vi "Create 4 In 4 Out Channel Resources.vi"(0 "common resources":T1={"sync pulse resources"={"sync pulse destination terminal"="", "sync100"="", "sync pulse source terminal"="", "imported sync pulse register"="", "generate sync pulse handshake"="", "enable sync pulse register"="", "sync pulse clock"=""}, "serial channel resources"={"sc 0"={"completed frames register"=""}, "sc 1"={"completed frames register"=""}, "sc 2"={"completed frames register"=""}, "sc 3"={"completed frames register"=""}, "sc 4"={"completed frames register"=""}, "sc 5"={"completed frames register"=""}, "sc 6"={"completed frames register"=""}, "sc 7"={"completed frames register"=""}}, "dram manager 0"={"DRAM class"=refnum, "process clock"="", "registers"={"configuration"={"write time slice"="", "request time slice"="", "DRAM arbiter config"="", "partition config"=""}, "reset"={"handshake"={"start.go"="", "start.go rcvd"="", "done.go"="", "done.go rcvd"=""}, "process"={"in"="", "out"=""}, "write"={"in"="", "out 0"="", "out 1"="", "out 2"="", "out 3"=""}, "read"={"in"="", "out 0"="", "out 1"="", "out 2"="", "out 3"=""}}, "status"={"partition full"=""}}, "FIFOs"={"write data"={"FIFO 0"="", "FIFO 1"="", "FIFO 2"="", "FIFO 3"=""}, "request metadata"={"FIFO"=""}, "read data VOQ"={"FIFO 0"="", "FIFO 1"="", "FIFO 2"="", "FIFO 3"=""}, "read data"={"FIFO 0"="", "FIFO 1"="", "FIFO 2"="", "FIFO 3"=""}}, "num active streams"=0.0, "max open read requests"=256}, "dram manager 1"={"DRAM class"=refnum, "process clock"="", "registers"={"configuration"={"write time slice"="", "request time slice"="", "DRAM arbiter config"="", "partition config"=""}, "reset"={"handshake"={"start.go"="", "start.go rcvd"="", "done.go"="", "done.go rcvd"=""}, "process"={"in"="", "out"=""}, "write"={"in"="", "out 0"="", "out 1"="", "out 2"="", "out 3"=""}, "read"={"in"="", "out 0"="", "out 1"="", "out 2"="", "out 3"=""}}, "status"={"partition full"=""}}, "FIFOs"={"write data"={"FIFO 0"="", "FIFO 1"="", "FIFO 2"="", "FIFO 3"=""}, "request metadata"={"FIFO"=""}, "read data VOQ"={"FIFO 0"="", "FIFO 1"="", "FIFO 2"="", "FIFO 3"=""}, "read data"={"FIFO 0"="", "FIFO 1"="", "FIFO 2"="", "FIFO 3"=""}}, "num active streams"=0.0, "max open read requests"=256}}, 5 "dram partition configs":T12[](array[typedef])=[{"first address"=0, "last address"=0}, {"first address"=0, "last address"=0}, {"first address"=0, "last address"=0}, {"first address"=0, "last address"=0}, {"first address"=0, "last address"=0}, {"first address"=0, "last address"=0}, {"first address"=0, "last address"=0}, {"first address"=0, "last address"=0}]) -> (4 "channel resources":T13)   [LabVIEW 2020, in "GettingStarted_Acq_Tap_148X_FPGA.lvlib"]
uses:
  GettingStarted_Acq_Tap_148X_FPGA.lvlib
  Types/4 In 4 Out Channel Resources.ctl
  <instrlib>/_niInstr/Memory/v1/FPGA/DRAM/niInstr Memory DRAM v1 FPGA.lvclass
  Types/Serial Input Channel Resources.ctl
  <instrlib>/FlexRIO/CSI-2/v2/FPGA/DRAM Manager/Private/DRAM Manager.ctl
  <instrlib>/FlexRIO/CSI-2/v2/FPGA/DRAM Manager/Private/Common/DRAM Manager Registers.ctl
  <instrlib>/FlexRIO/CSI-2/v2/FPGA/DRAM Manager/Private/Common/Handshake Registers.ctl
  <instrlib>/FlexRIO/CSI-2/v2/FPGA/DRAM Manager/Private/Common/DRAM Manager FIFOs.ctl
  <instrlib>/FlexRIO/CSI-2/v2/FPGA/DRAM Manager/Private/Common/Write Data FIFO Ref.ctl
  <instrlib>/FlexRIO/CSI-2/v2/FPGA/DRAM Manager/Private/Common/Read Request Metadata FIFO Ref.ctl
  <instrlib>/FlexRIO/CSI-2/v2/FPGA/DRAM Manager/Private/Common/Read Data FIFO Ref.ctl
  Types/Serial Input Channel IO.ctl
  Types/Serial Input Channel IO 32b.ctl
  Types/Serial Input Channel IO 64b.ctl
  Common/Types/I2C IO.ctl
  Types/Serial Ouput Channel Resources.ctl
  Common/Types/Serial Output Channel IO.ctl
  Common/Types/Serial Output Channel IO 32b.ctl
  Common/Types/Serial Output Channel IO 64b.ctl
  <instrlib>/FlexRIO/CSI-2/v2/FPGA/DRAM Manager/Public/Partition Range.ctl
  Common/Types/Common Resources.ctl
  <instrlib>/FlexRIO/CSI-2/v2/FPGA/Types/Sync Pulse Resources.ctl
  Common/Types/Serial Channel Resources.ctl
  Common/Types/Single Serial Channel Resources.ctl
  <instrlib>/FlexRIO/CSI-2/v2/FPGA/DRAM Manager/DRAM Manager v2.lvlib
  Common/GettingStarted_Common_148X_FPGA.lvlib
  <instrlib>/FlexRIO/CSI-2/v2/FPGA/NI CSI-2 API FPGA v2.lvlib
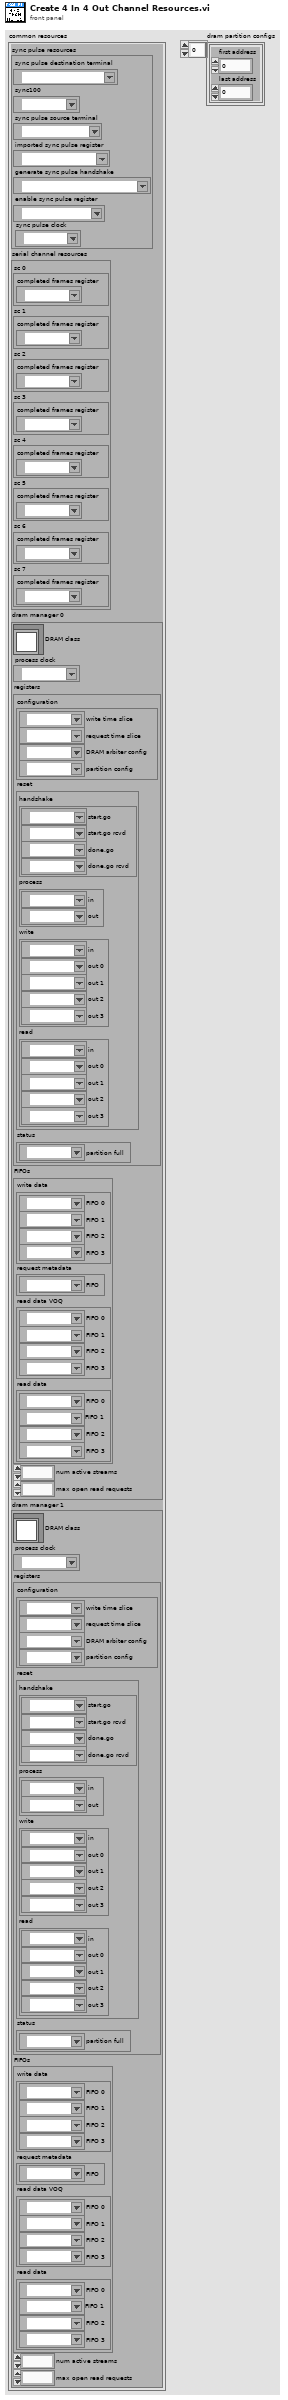
[diagram p1: front panel]
types:
  T1 = typedef "GettingStarted_Common_148X_FPGA.lvlib/Common Resources.ctl" = cluster{"sync pulse resources":T2, "serial channel resources":T3, "dram manager 0":T5, "dram manager 1":T5}
  T2 = typedef "NI CSI-2 API FPGA v2.lvlib/Sync Pulse Resources.ctl" = cluster{"sync pulse destination terminal":refnum<k21>, "sync100":refnum<k21>, "sync pulse source terminal":refnum<k21>, "imported sync pulse register":refnum<k21>, "generate sync pulse handshake":refnum<k21>, "enable sync pulse register":refnum<k21>, "sync pulse clock":refnum<k21>}
  T3 = typedef "GettingStarted_Common_148X_FPGA.lvlib/Serial Channel Resources.ctl" = cluster{"sc 0":T4, "sc 1":T4, "sc 2":T4, "sc 3":T4, "sc 4":T4, "sc 5":T4, "sc 6":T4, "sc 7":T4}
  T4 = typedef "GettingStarted_Common_148X_FPGA.lvlib/Single Serial Channel Resources.ctl" = cluster{"completed frames register":refnum<k21>}
  T5 = typedef "DRAM Manager v2.lvlib/DRAM Manager.ctl" = cluster{"DRAM class":refnum<class "niInstr Memory DRAM v1 FPGA.lvclass">, "process clock":refnum<k21>, "registers":T6, "FIFOs":T8, "num active streams":fxp<+,3,3>, "max open read requests":u16}
  T6 = typedef "DRAM Manager v2.lvlib/DRAM Manager Registers.ctl" = cluster{"configuration":cluster{"write time slice":refnum<k21>, "request time slice":refnum<k21>, "DRAM arbiter config":refnum<k21>, "partition config":refnum<k21>}, "reset":cluster{"handshake":T7, "process":cluster{"in":refnum<k21>, "out":refnum<k21>}, "write":cluster{"in":refnum<k21>, "out 0":refnum<k21>, "out 1":refnum<k21>, "out 2":refnum<k21>, "out 3":refnum<k21>}, "read":cluster{"in":refnum<k21>, "out 0":refnum<k21>, "out 1":refnum<k21>, "out 2":refnum<k21>, "out 3":refnum<k21>}}, "status":cluster{"partition full":refnum<k21>}}
  T7 = typedef "DRAM Manager v2.lvlib/Handshake Registers.ctl" = cluster{"start.go":refnum<k21>, "start.go rcvd":refnum<k21>, "done.go":refnum<k21>, "done.go rcvd":refnum<k21>}
  T8 = typedef "DRAM Manager v2.lvlib/DRAM Manager FIFOs.ctl" = cluster{"write data":cluster{"FIFO 0":T9, "FIFO 1":T9, "FIFO 2":T9, "FIFO 3":T9}, "request metadata":cluster{"FIFO":T10}, "read data VOQ":cluster{"FIFO 0":T11, "FIFO 1":T11, "FIFO 2":T11, "FIFO 3":T11}, "read data":cluster{"FIFO 0":T11, "FIFO 1":T11, "FIFO 2":T11, "FIFO 3":T11}}
  T9 = typedef "DRAM Manager v2.lvlib/Write Data FIFO Ref.ctl" = refnum<k21>
  T10 = typedef "DRAM Manager v2.lvlib/Read Request Metadata FIFO Ref.ctl" = refnum<k21>
  T11 = typedef "DRAM Manager v2.lvlib/Read Data FIFO Ref.ctl" = refnum<k21>
  T12 = typedef "DRAM Manager v2.lvlib/Partition Range.ctl" = cluster{"first address":u32, "last address":u32}
  T13 = typedef "GettingStarted_Acq_Tap_148X_FPGA.lvlib/4 In 4 Out Channel Resources.ctl" = cluster{"si 0 resources":T14, "si 1 resources":T14, "si 2 resources":T14, "si 3 resources":T14, "so 0 resources":T19, "so 1 resources":T19, "so 2 resources":T19, "so 3 resources":T19}
  T14 = typedef "GettingStarted_Acq_Tap_148X_FPGA.lvlib/Serial Input Channel Resources.ctl" = cluster{"dram manager":T5, "csi-2 input io":T15, "serial input channel instance":u8, "dram stream id":fxp<+,2,2>, "i2c io":T18}
  T15 = typedef "GettingStarted_Acq_Tap_148X_FPGA.lvlib/Serial Input Channel IO.ctl" = cluster{"32b":T16, "64b":T17, "csi-2 axi stream tlast":refnum<k21>, "csi-2 axi stream tvalid":refnum<k21>}
  T16 = typedef "GettingStarted_Acq_Tap_148X_FPGA.lvlib/Serial Input Channel IO 32b.ctl" = cluster{"csi-2 axi stream tdata":refnum<k21>, "csi-2 axi stream raw tdata":refnum<k21>, "csi-2 axi stream tuser":refnum<k21>}
  T17 = typedef "GettingStarted_Acq_Tap_148X_FPGA.lvlib/Serial Input Channel IO 64b.ctl" = cluster{"csi-2 axi stream tdata":refnum<k21>, "csi-2 axi stream raw tdata":refnum<k21>, "csi-2 axi stream tuser":refnum<k21>}
  T18 = typedef "GettingStarted_Common_148X_FPGA.lvlib/I2C IO.ctl" = cluster{"sda input":refnum<k21>, "sda output enable":refnum<k21>, "scl input":refnum<k21>, "scl output enable":refnum<k21>}
  T19 = typedef "GettingStarted_Acq_Tap_148X_FPGA.lvlib/Serial Ouput Channel Resources.ctl" = cluster{"csi-2 output io":T20, "i2c io":T18}
  T20 = typedef "GettingStarted_Common_148X_FPGA.lvlib/Serial Output Channel IO.ctl" = cluster{"32b":T21, "64b":T22, "csi-2 axi stream tready":refnum<k21>, "csi-2 axi stream tvalid":refnum<k21>, "csi-2 axi stream tlast":refnum<k21>, "num packets in tx fifo":refnum<k21>, "ready to transmit packet":refnum<k21>, "transmit packet done":refnum<k21>, "transmit packet":refnum<k21>}
  T21 = typedef "GettingStarted_Common_148X_FPGA.lvlib/Serial Output Channel IO 32b.ctl" = cluster{"csi-2 axi stream tdata":refnum<k21>, "csi-2 axi stream tuser":refnum<k21>}
  T22 = typedef "GettingStarted_Common_148X_FPGA.lvlib/Serial Output Channel IO 64b.ctl" = cluster{"csi-2 axi stream tdata":refnum<k21>, "csi-2 axi stream tuser":refnum<k21>}
  T23 = cluster{"serial input 0 csi-2 io":T15, "serial input 1 csi-2 io":T15, "serial input 2 csi-2 io":T15, "serial input 3 csi-2 io":T15}
  T24 = cluster{"serial input 0 i2c io":T18, "serial input 1 i2c io":T18, "serial input 2 i2c io":T18, "serial input 3 i2c io":T18}
  T25 = cluster{"serial output 0 io":T20, "serial output 1 io":T20, "serial output 2 io":T20, "serial output 3 io":T20}
  T26 = cluster{"serial output 2 i2c io":T18, "serial output 1 i2c io":T18, "serial output 0 i2c io":T18, "serial output 3 i2c io":T18}
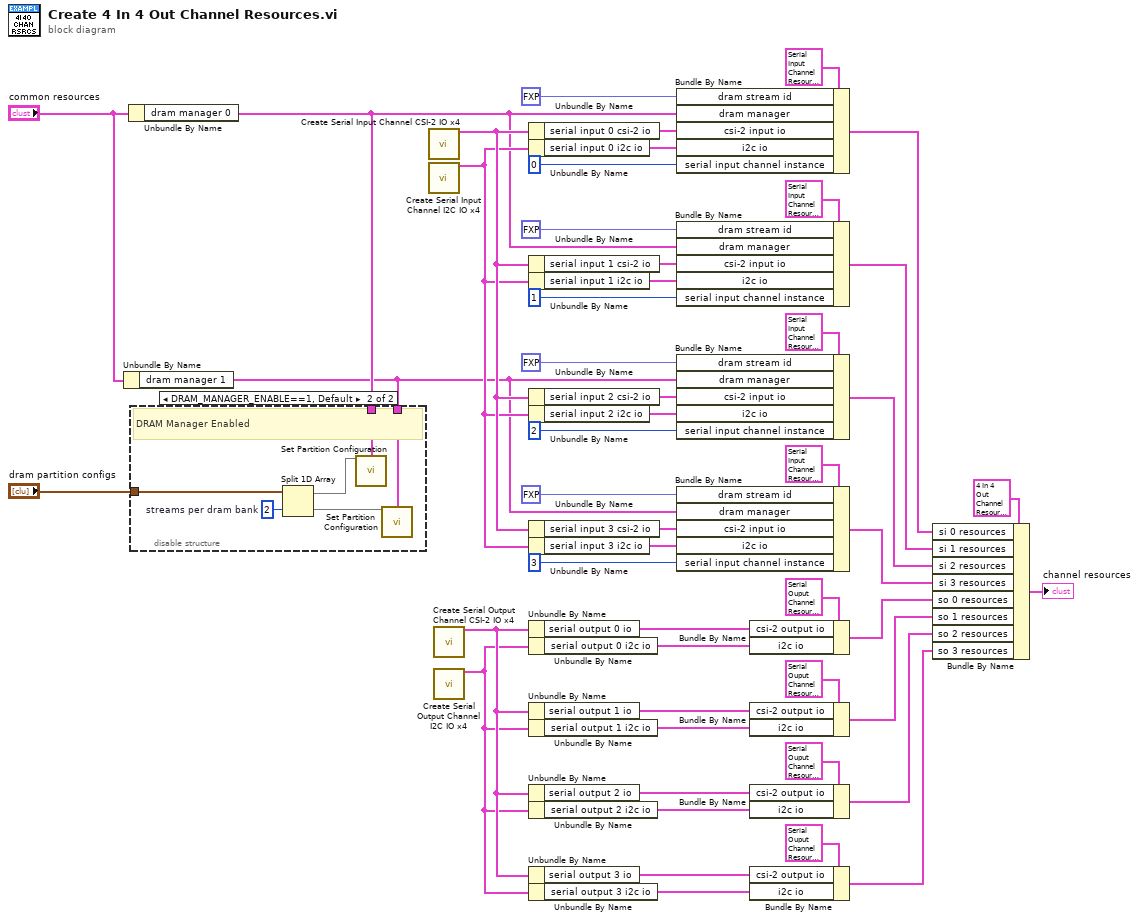
[diagram p0: block diagram]
diagram:
  n1 = Unbundle By Name("common resources") -> ("dram manager 1"=w3:T5)
  n2 = Unbundle By Name("common resources") -> ("dram manager 0"=w4:T5)
  n3 = disable-structure shown="DRAM_MANAGER_ENABLE==1, Default" {
    disable-tunnel: w4 -> [_ w53]
    disable-tunnel: w3 -> [_ w52]
    disable-tunnel: "dram partition configs" -> [_ w51]
    frame condition #0 {
      # "DRAM Manager Disabled"
    }
    frame condition #1 (active) {
      w56 = 2  # streams per dram bank
      # "DRAM Manager Enabled"
      n4 = Split 1D Array(array=w51, index=w56) -> (first subarray=w55:T12[], second subarray=w54:T12[])
      n5 = call <instrlib>:"Set Partition Configuration.vi"("partition config"=w55, "DRAM manager"=w53) -> ()  [unwired: 14 in]
      n6 = call <instrlib>:"Set Partition Configuration.vi"("partition config"=w54, "DRAM manager"=w52) -> ()  [unwired: 14 in]
    }
  }
  n7 = call "Create Serial Input Channel CSI-2 IO x4.vi"() -> ("serial input csi-2 io x4"=w20:T23)  [unwired: 15 in]
  n8 = call "Create Serial Input Channel I2C IO x4.vi"() -> ("serial input channel i2c io x4"=w5:T24)  [unwired: 15 in]
  n9 = call "Create Serial Output Channel CSI-2 IO x4.vi"() -> ("serial output channel csi-2 io x4 2"=w15:T25)  [unwired: 15 in]
  n10 = call "Create Serial Output Channel I2C IO x4.vi"() -> ("serial output channel i2c io x4"=w10:T26)  [unwired: 15 in]
  n11 = Unbundle By Name(w20) -> ("serial input 0 csi-2 io"=w24:T15)
  n12 = Unbundle By Name(w5) -> ("serial input 0 i2c io"=w6:T18)
  n13 = Unbundle By Name(w20) -> ("serial input 1 csi-2 io"=w23:T15)
  n14 = Unbundle By Name(w5) -> ("serial input 1 i2c io"=w7:T18)
  n15 = Unbundle By Name(w20) -> ("serial input 2 csi-2 io"=w22:T15)
  n16 = Unbundle By Name(w5) -> ("serial input 2 i2c io"=w8:T18)
  n17 = Unbundle By Name(w20) -> ("serial input 3 csi-2 io"=w21:T15)
  n18 = Unbundle By Name(w5) -> ("serial input 3 i2c io"=w9:T18)
  n19 = Unbundle By Name(w15) -> ("serial output 0 io"=w19:T20)
  n20 = Unbundle By Name(w10) -> ("serial output 0 i2c io"=w14:T18)
  n21 = Unbundle By Name(w15) -> ("serial output 1 io"=w18:T20)
  n22 = Unbundle By Name(w10) -> ("serial output 1 i2c io"=w13:T18)
  n23 = Unbundle By Name(w15) -> ("serial output 2 io"=w17:T20)
  n24 = Unbundle By Name(w10) -> ("serial output 2 i2c io"=w12:T18)
  n25 = Unbundle By Name(w15) -> ("serial output 3 io"=w16:T20)
  n26 = Unbundle By Name(w10) -> ("serial output 3 i2c io"=w11:T18)
  n27 = Bundle By Name(cluster=T14 {"dram manager"={"DRAM class"=refnum, "process clock"="", "registers"={"configuration"={"write time slice"="", "request time slice"="", "DRAM arbiter config"="", "partition config"=""}, "reset"={"handshake"={"start.go"="", "start.go rcvd"="", "done.go"="", "done.go rcvd"=""}, "process"={"in"="", "out"=""}, "write"={"in"="", "out 0"="", "out 1"="", "out 2"="", "out 3"=""}, "read"={"in"="", "out 0"="", "out 1"="", "out 2"="", "out 3"=""}}, "status"={"partition full"=""}}, "FIFOs"={"write data"={"FIFO 0"="", "FIFO 1"="", "FIFO 2"="", "FIFO 3"=""}, "request metadata"={"FIFO"=""}, "read data VOQ"={"FIFO 0"="", "FIFO 1"="", "FIFO 2"="", "FIFO 3"=""}, "read data"={"FIFO 0"="", "FIFO 1"="", "FIFO 2"="", "FIFO 3"=""}}, "num active streams"=0.0, "max open read requests"=0}, "csi-2 input io"={"32b"={"csi-2 axi stream tdata"="", "csi-2 axi stream raw tdata"="", "csi-2 axi stream tuser"=""}, "64b"={"csi-2 axi stream tdata"="", "csi-2 axi stream raw tdata"="", "csi-2 axi stream tuser"=""}, "csi-2 axi stream tlast"="", "csi-2 axi stream tvalid"=""}, "serial input channel instance"=0, "dram stream id"=0.0, "i2c io"={"sda input"="", "sda output enable"="", "scl input"="", "scl output enable"=""}} ("si 0 resources"), "dram stream id"=fxp<+,2,2> 0.0, "dram manager"=w4, "csi-2 input io"=w24, "i2c io"=w6, "serial input channel instance"=u8 0) -> (w50:T14)
  n28 = Bundle By Name(cluster=T14 {"dram manager"={"DRAM class"=refnum, "process clock"="", "registers"={"configuration"={"write time slice"="", "request time slice"="", "DRAM arbiter config"="", "partition config"=""}, "reset"={"handshake"={"start.go"="", "start.go rcvd"="", "done.go"="", "done.go rcvd"=""}, "process"={"in"="", "out"=""}, "write"={"in"="", "out 0"="", "out 1"="", "out 2"="", "out 3"=""}, "read"={"in"="", "out 0"="", "out 1"="", "out 2"="", "out 3"=""}}, "status"={"partition full"=""}}, "FIFOs"={"write data"={"FIFO 0"="", "FIFO 1"="", "FIFO 2"="", "FIFO 3"=""}, "request metadata"={"FIFO"=""}, "read data VOQ"={"FIFO 0"="", "FIFO 1"="", "FIFO 2"="", "FIFO 3"=""}, "read data"={"FIFO 0"="", "FIFO 1"="", "FIFO 2"="", "FIFO 3"=""}}, "num active streams"=0.0, "max open read requests"=0}, "csi-2 input io"={"32b"={"csi-2 axi stream tdata"="", "csi-2 axi stream raw tdata"="", "csi-2 axi stream tuser"=""}, "64b"={"csi-2 axi stream tdata"="", "csi-2 axi stream raw tdata"="", "csi-2 axi stream tuser"=""}, "csi-2 axi stream tlast"="", "csi-2 axi stream tvalid"=""}, "serial input channel instance"=0, "dram stream id"=0.0, "i2c io"={"sda input"="", "sda output enable"="", "scl input"="", "scl output enable"=""}} ("si 0 resources"), "dram stream id"=fxp<+,2,2> 1.0, "dram manager"=w4, "csi-2 input io"=w23, "i2c io"=w7, "serial input channel instance"=u8 1) -> (w49:T14)
  n29 = Bundle By Name(cluster=T14 {"dram manager"={"DRAM class"=refnum, "process clock"="", "registers"={"configuration"={"write time slice"="", "request time slice"="", "DRAM arbiter config"="", "partition config"=""}, "reset"={"handshake"={"start.go"="", "start.go rcvd"="", "done.go"="", "done.go rcvd"=""}, "process"={"in"="", "out"=""}, "write"={"in"="", "out 0"="", "out 1"="", "out 2"="", "out 3"=""}, "read"={"in"="", "out 0"="", "out 1"="", "out 2"="", "out 3"=""}}, "status"={"partition full"=""}}, "FIFOs"={"write data"={"FIFO 0"="", "FIFO 1"="", "FIFO 2"="", "FIFO 3"=""}, "request metadata"={"FIFO"=""}, "read data VOQ"={"FIFO 0"="", "FIFO 1"="", "FIFO 2"="", "FIFO 3"=""}, "read data"={"FIFO 0"="", "FIFO 1"="", "FIFO 2"="", "FIFO 3"=""}}, "num active streams"=0.0, "max open read requests"=0}, "csi-2 input io"={"32b"={"csi-2 axi stream tdata"="", "csi-2 axi stream raw tdata"="", "csi-2 axi stream tuser"=""}, "64b"={"csi-2 axi stream tdata"="", "csi-2 axi stream raw tdata"="", "csi-2 axi stream tuser"=""}, "csi-2 axi stream tlast"="", "csi-2 axi stream tvalid"=""}, "serial input channel instance"=0, "dram stream id"=0.0, "i2c io"={"sda input"="", "sda output enable"="", "scl input"="", "scl output enable"=""}} ("si 0 resources"), "dram stream id"=fxp<+,2,2> 0.0, "dram manager"=w3, "csi-2 input io"=w22, "i2c io"=w8, "serial input channel instance"=u8 2) -> (w48:T14)
  n30 = Bundle By Name(cluster=T14 {"dram manager"={"DRAM class"=refnum, "process clock"="", "registers"={"configuration"={"write time slice"="", "request time slice"="", "DRAM arbiter config"="", "partition config"=""}, "reset"={"handshake"={"start.go"="", "start.go rcvd"="", "done.go"="", "done.go rcvd"=""}, "process"={"in"="", "out"=""}, "write"={"in"="", "out 0"="", "out 1"="", "out 2"="", "out 3"=""}, "read"={"in"="", "out 0"="", "out 1"="", "out 2"="", "out 3"=""}}, "status"={"partition full"=""}}, "FIFOs"={"write data"={"FIFO 0"="", "FIFO 1"="", "FIFO 2"="", "FIFO 3"=""}, "request metadata"={"FIFO"=""}, "read data VOQ"={"FIFO 0"="", "FIFO 1"="", "FIFO 2"="", "FIFO 3"=""}, "read data"={"FIFO 0"="", "FIFO 1"="", "FIFO 2"="", "FIFO 3"=""}}, "num active streams"=0.0, "max open read requests"=0}, "csi-2 input io"={"32b"={"csi-2 axi stream tdata"="", "csi-2 axi stream raw tdata"="", "csi-2 axi stream tuser"=""}, "64b"={"csi-2 axi stream tdata"="", "csi-2 axi stream raw tdata"="", "csi-2 axi stream tuser"=""}, "csi-2 axi stream tlast"="", "csi-2 axi stream tvalid"=""}, "serial input channel instance"=0, "dram stream id"=0.0, "i2c io"={"sda input"="", "sda output enable"="", "scl input"="", "scl output enable"=""}} ("si 0 resources"), "dram stream id"=fxp<+,2,2> 1.0, "dram manager"=w3, "csi-2 input io"=w21, "i2c io"=w9, "serial input channel instance"=u8 3) -> (w47:T14)
  n31 = Bundle By Name(cluster=T19 {"csi-2 output io"={"32b"={"csi-2 axi stream tdata"="", "csi-2 axi stream tuser"=""}, "64b"={"csi-2 axi stream tdata"="", "csi-2 axi stream tuser"=""}, "csi-2 axi stream tready"="", "csi-2 axi stream tvalid"="", "csi-2 axi stream tlast"="", "num packets in tx fifo"="", "ready to transmit packet"="", "transmit packet done"="", "transmit packet"=""}, "i2c io"={"sda input"="", "sda output enable"="", "scl input"="", "scl output enable"=""}} ("so 0 resources"), "csi-2 output io"=w19, "i2c io"=w14) -> (w46:T19)
  n32 = Bundle By Name(cluster=T19 {"csi-2 output io"={"32b"={"csi-2 axi stream tdata"="", "csi-2 axi stream tuser"=""}, "64b"={"csi-2 axi stream tdata"="", "csi-2 axi stream tuser"=""}, "csi-2 axi stream tready"="", "csi-2 axi stream tvalid"="", "csi-2 axi stream tlast"="", "num packets in tx fifo"="", "ready to transmit packet"="", "transmit packet done"="", "transmit packet"=""}, "i2c io"={"sda input"="", "sda output enable"="", "scl input"="", "scl output enable"=""}} ("so 0 resources"), "csi-2 output io"=w18, "i2c io"=w13) -> (w45:T19)
  n33 = Bundle By Name(cluster=T19 {"csi-2 output io"={"32b"={"csi-2 axi stream tdata"="", "csi-2 axi stream tuser"=""}, "64b"={"csi-2 axi stream tdata"="", "csi-2 axi stream tuser"=""}, "csi-2 axi stream tready"="", "csi-2 axi stream tvalid"="", "csi-2 axi stream tlast"="", "num packets in tx fifo"="", "ready to transmit packet"="", "transmit packet done"="", "transmit packet"=""}, "i2c io"={"sda input"="", "sda output enable"="", "scl input"="", "scl output enable"=""}} ("so 0 resources"), "csi-2 output io"=w17, "i2c io"=w12) -> (w44:T19)
  n34 = Bundle By Name(cluster=T19 {"csi-2 output io"={"32b"={"csi-2 axi stream tdata"="", "csi-2 axi stream tuser"=""}, "64b"={"csi-2 axi stream tdata"="", "csi-2 axi stream tuser"=""}, "csi-2 axi stream tready"="", "csi-2 axi stream tvalid"="", "csi-2 axi stream tlast"="", "num packets in tx fifo"="", "ready to transmit packet"="", "transmit packet done"="", "transmit packet"=""}, "i2c io"={"sda input"="", "sda output enable"="", "scl input"="", "scl output enable"=""}} ("so 0 resources"), "csi-2 output io"=w16, "i2c io"=w11) -> (w43:T19)
  n35 = Bundle By Name(cluster=T13 {"si 0 resources"={"dram manager"={"DRAM class"=refnum, "process clock"="", "registers"={"configuration"={"write time slice"="", "request time slice"="", "DRAM arbiter config"="", "partition config"=""}, "reset"={"handshake"={"start.go"="", "start.go rcvd"="", "done.go"="", "done.go rcvd"=""}, "process"={"in"="", "out"=""}, "write"={"in"="", "out 0"="", "out 1"="", "out 2"="", "out 3"=""}, "read"={"in"="", "out 0"="", "out 1"="", "out 2"="", "out 3"=""}}, "status"={"partition full"=""}}, "FIFOs"={"write data"={"FIFO 0"="", "FIFO 1"="", "FIFO 2"="", "FIFO 3"=""}, "request metadata"={"FIFO"=""}, "read data VOQ"={"FIFO 0"="", "FIFO 1"="", "FIFO 2"="", "FIFO 3"=""}, "read data"={"FIFO 0"="", "FIFO 1"="", "FIFO 2"="", "FIFO 3"=""}}, "num active streams"=0.0, "max open read requests"=0}, "csi-2 input io"={"32b"={"csi-2 axi stream tdata"="", "csi-2 axi stream raw tdata"="", "csi-2 axi stream tuser"=""}, "64b"={"csi-2 axi stream tdata"="", "csi-2 axi stream raw tdata"="", "csi-2 axi stream tuser"=""}, "csi-2 axi stream tlast"="", "csi-2 axi stream tvalid"=""}, "serial input channel instance"=0, "dram stream id"=0.0, "i2c io"={"sda input"="", "sda output enable"="", "scl input"="", "scl output enable"=""}}, "si 1 resources"={"dram manager"={"DRAM class"=refnum, "process clock"="", "registers"={"configuration"={"write time slice"="", "request time slice"="", "DRAM arbiter config"="", "partition config"=""}, "reset"={"handshake"={"start.go"="", "start.go rcvd"="", "done.go"="", "done.go rcvd"=""}, "process"={"in"="", "out"=""}, "write"={"in"="", "out 0"="", "out 1"="", "out 2"="", "out 3"=""}, "read"={"in"="", "out 0"="", "out 1"="", "out 2"="", "out 3"=""}}, "status"={"partition full"=""}}, "FIFOs"={"write data"={"FIFO 0"="", "FIFO 1"="", "FIFO 2"="", "FIFO 3"=""}, "request metadata"={"FIFO"=""}, "read data VOQ"={"FIFO 0"="", "FIFO 1"="", "FIFO 2"="", "FIFO 3"=""}, "read data"={"FIFO 0"="", "FIFO 1"="", "FIFO 2"="", "FIFO 3"=""}}, "num active streams"=0.0, "max open read requests"=0}, "csi-2 input io"={"32b"={"csi-2 axi stream tdata"="", "csi-2 axi stream raw tdata"="", "csi-2 axi stream tuser"=""}, "64b"={"csi-2 axi stream tdata"="", "csi-2 axi stream raw tdata"="", "csi-2 axi stream tuser"=""}, "csi-2 axi stream tlast"="", "csi-2 axi stream tvalid"=""}, "serial input channel instance"=0, "dram stream id"=0.0, "i2c io"={"sda input"="", "sda output enable"="", "scl input"="", "scl output enable"=""}}, "si 2 resources"={"dram manager"={"DRAM class"=refnum, "process clock"="", "registers"={"configuration"={"write time slice"="", "request time slice"="", "DRAM arbiter config"="", "partition config"=""}, "reset"={"handshake"={"start.go"="", "start.go rcvd"="", "done.go"="", "done.go rcvd"=""}, "process"={"in"="", "out"=""}, "write"={"in"="", "out 0"="", "out 1"="", "out 2"="", "out 3"=""}, "read"={"in"="", "out 0"="", "out 1"="", "out 2"="", "out 3"=""}}, "status"={"partition full"=""}}, "FIFOs"={"write data"={"FIFO 0"="", "FIFO 1"="", "FIFO 2"="", "FIFO 3"=""}, "request metadata"={"FIFO"=""}, "read data VOQ"={"FIFO 0"="", "FIFO 1"="", "FIFO 2"="", "FIFO 3"=""}, "read data"={"FIFO 0"="", "FIFO 1"="", "FIFO 2"="", "FIFO 3"=""}}, "num active streams"=0.0, "max open read requests"=0}, "csi-2 input io"={"32b"={"csi-2 axi stream tdata"="", "csi-2 axi stream raw tdata"="", "csi-2 axi stream tuser"=""}, "64b"={"csi-2 axi stream tdata"="", "csi-2 axi stream raw tdata"="", "csi-2 axi stream tuser"=""}, "csi-2 axi stream tlast"="", "csi-2 axi stream tvalid"=""}, "serial input channel instance"=0, "dram stream id"=0.0, "i2c io"={"sda input"="", "sda output enable"="", "scl input"="", "scl output enable"=""}}, "si 3 resources"={"dram manager"={"DRAM class"=refnum, "process clock"="", "registers"={"configuration"={"write time slice"="", "request time slice"="", "DRAM arbiter config"="", "partition config"=""}, "reset"={"handshake"={"start.go"="", "start.go rcvd"="", "done.go"="", "done.go rcvd"=""}, "process"={"in"="", "out"=""}, "write"={"in"="", "out 0"="", "out 1"="", "out 2"="", "out 3"=""}, "read"={"in"="", "out 0"="", "out 1"="", "out 2"="", "out 3"=""}}, "status"={"partition full"=""}}, "FIFOs"={"write data"={"FIFO 0"="", "FIFO 1"="", "FIFO 2"="", "FIFO 3"=""}, "request metadata"={"FIFO"=""}, "read data VOQ"={"FIFO 0"="", "FIFO 1"="", "FIFO 2"="", "FIFO 3"=""}, "read data"={"FIFO 0"="", "FIFO 1"="", "FIFO 2"="", "FIFO 3"=""}}, "num active streams"=0.0, "max open read requests"=0}, "csi-2 input io"={"32b"={"csi-2 axi stream tdata"="", "csi-2 axi stream raw tdata"="", "csi-2 axi stream tuser"=""}, "64b"={"csi-2 axi stream tdata"="", "csi-2 axi stream raw tdata"="", "csi-2 axi stream tuser"=""}, "csi-2 axi stream tlast"="", "csi-2 axi stream tvalid"=""}, "serial input channel instance"=0, "dram stream id"=0.0, "i2c io"={"sda input"="", "sda output enable"="", "scl input"="", "scl output enable"=""}}, "so 0 resources"={"csi-2 output io"={"32b"={"csi-2 axi stream tdata"="", "csi-2 axi stream tuser"=""}, "64b"={"csi-2 axi stream tdata"="", "csi-2 axi stream tuser"=""}, "csi-2 axi stream tready"="", "csi-2 axi stream tvalid"="", "csi-2 axi stream tlast"="", "num packets in tx fifo"="", "ready to transmit packet"="", "transmit packet done"="", "transmit packet"=""}, "i2c io"={"sda input"="", "sda output enable"="", "scl input"="", "scl output enable"=""}}, "so 1 resources"={"csi-2 output io"={"32b"={"csi-2 axi stream tdata"="", "csi-2 axi stream tuser"=""}, "64b"={"csi-2 axi stream tdata"="", "csi-2 axi stream tuser"=""}, "csi-2 axi stream tready"="", "csi-2 axi stream tvalid"="", "csi-2 axi stream tlast"="", "num packets in tx fifo"="", "ready to transmit packet"="", "transmit packet done"="", "transmit packet"=""}, "i2c io"={"sda input"="", "sda output enable"="", "scl input"="", "scl output enable"=""}}, "so 2 resources"={"csi-2 output io"={"32b"={"csi-2 axi stream tdata"="", "csi-2 axi stream tuser"=""}, "64b"={"csi-2 axi stream tdata"="", "csi-2 axi stream tuser"=""}, "csi-2 axi stream tready"="", "csi-2 axi stream tvalid"="", "csi-2 axi stream tlast"="", "num packets in tx fifo"="", "ready to transmit packet"="", "transmit packet done"="", "transmit packet"=""}, "i2c io"={"sda input"="", "sda output enable"="", "scl input"="", "scl output enable"=""}}, "so 3 resources"={"csi-2 output io"={"32b"={"csi-2 axi stream tdata"="", "csi-2 axi stream tuser"=""}, "64b"={"csi-2 axi stream tdata"="", "csi-2 axi stream tuser"=""}, "csi-2 axi stream tready"="", "csi-2 axi stream tvalid"="", "csi-2 axi stream tlast"="", "num packets in tx fifo"="", "ready to transmit packet"="", "transmit packet done"="", "transmit packet"=""}, "i2c io"={"sda input"="", "sda output enable"="", "scl input"="", "scl output enable"=""}}}, "si 0 resources"=w50, "si 1 resources"=w49, "si 2 resources"=w48, "si 3 resources"=w47, "so 0 resources"=w46, "so 1 resources"=w45, "so 2 resources"=w44, "so 3 resources"=w43) -> (→"channel resources":T13)
